vi "Main_DC.vi"() -> ()   [LabVIEW 2014]
uses:
  <vilib>/myRIO/Instrument Drivers/Utilities/Utilities.lvlib
  <vilib>/myRIO/Express VI/Onboard IO/Encoder/Encoder Express VI.xnode
  <vilib>/myRIO/Instrument Drivers/Onboard IO/Encoder/vis/Read.vi
  <vilib>/myRIO/Instrument Drivers/Onboard IO/Encoder/Encoder.lvlib
  <vilib>/myRIO/Common/Instrument Driver Framework/myRIO v1.0/Encoder/typedefs/Encoder Signal Mode.ctl
  <vilib>/myRIO/Common/Instrument Driver Framework/myRIO v1.0/Encoder/typedefs/Encoder Channels Enum.ctl
  <vilib>/myRIO/Common/Instrument Driver Framework/Utilities/typedefs/Generic FPGA Reference.ctl
  <vilib>/myRIO/Common/Instrument Driver Framework/Utilities/typedefs/myRIO v1.0 Reference.ctl
  <vilib>/myRIO/Common/Instrument Driver Framework/Utilities/typedefs/Hardware Version Enum.ctl
  <vilib>/myRIO/Common/Instrument Driver Framework/Utilities/typedefs/myRIO Generic Hardware Reference.ctl
  <vilib>/myRIO/Instrument Drivers/Onboard IO/Encoder/typedefs/Encoder Reference.ctl
  <vilib>/myRIO/Instrument Drivers/Onboard IO/Encoder/vis/myRIO Encoder Open.xnode
  <vilib>/myRIO/Common/Instrument Driver Framework/Utilities/vis/Is FPGA Ref Available.vi
  <vilib>/myRIO/Common/Instrument Driver Framework/myRIO v1.0/Encoder/vis/myRIO v1.1 Open Encoder.vi
  <vilib>/myRIO/Common/Instrument Driver Framework/myRIO v1.0/Encoder/vis/myRIO v1.0 Configure Encoder.vi
  <vilib>/myRIO/Common/Instrument Driver Framework/myRIO v1.0/Encoder/typedefs/Encoder Configuration v1.0.ctl
  <vilib>/userdefined/High Color/nirio_resource_hc.ctl
  <vilib>/myRIO/Common/Instrument Driver Framework/myRIO v1.0/Encoder/typedefs/Encoder Count Direction Enum.ctl
panel:
  in  "PWM freq [Hz]":dbl(slide)=10000.0 scale=5000.0..20000.0
  in  "PWM duty  [%]":dbl(slide) scale=-99.0..99.0
  in  "PWM duty  [%]":dbl(slide) scale=-99.0..99.0
  in  "PWM freq [Hz]":dbl(slide)=10000.0 scale=5000.0..20000.0
  in  "Reset Counter":bool
  out "Counter Direction":T1
  out "Counter Value":i32
  in  "[ESC]":bool
  # "DC Motor Testing"
  # "MOTOR 1"
  # "MOTOR 2"
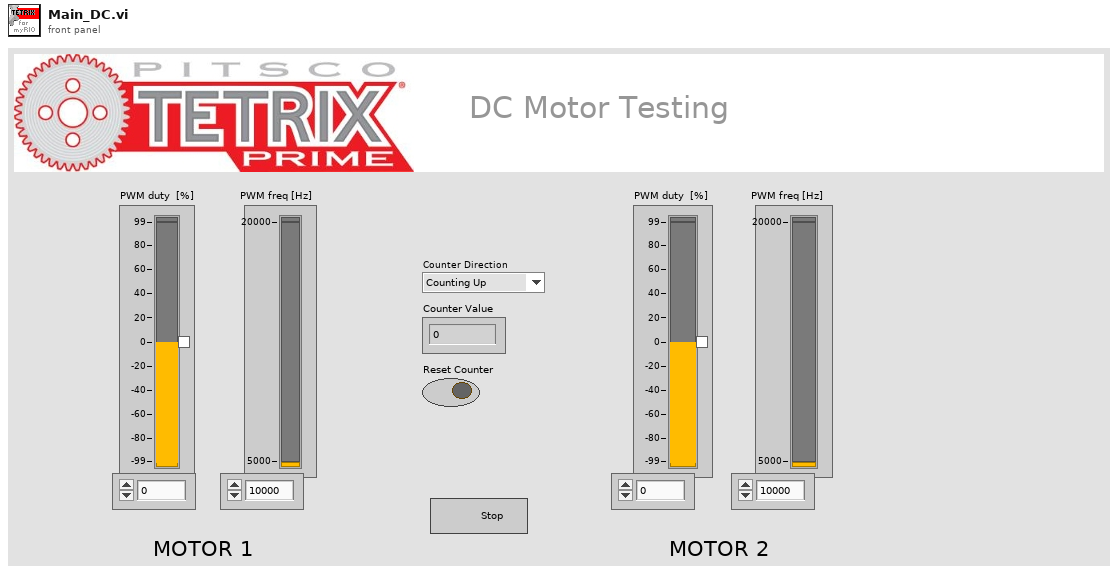
[diagram p1: front panel]
types:
  T1 = typedef "Encoder Count Direction Enum.ctl" = enum16{"Counting Up", "Counting Down"}
  T2 = typedef "Encoder.lvlib/Encoder Reference.ctl" = cluster{"myRIO Reference":T3, "Encoder Channels Enum":T7}
  T3 = typedef "myRIO Generic Hardware Reference.ctl" = cluster{"myRIO Model":T4, "myRIO Hardware Reference":T5}
  T4 = typedef "Hardware Version Enum.ctl" = enum16{"Unknown", "myRIO-1900", "myRIO-1950"}
  T5 = typedef "myRIO v1.0 Reference.ctl" = cluster{"Generic FPGA Reference":T6, "Allow multiple opens":bool}
  T6 = typedef "Generic FPGA Reference.ctl" = refnum<k20>
  T7 = typedef "Encoder Channels Enum.ctl" = enum16{"Not Connected", "C/ENC0", "C/ENC1", "A/ENC", "B/ENC"}
  T8 = typedef "Encoder Signal Mode.ctl" = enum16{"Quadrature phase signal", "Step and direction signal"}
  T9 = typedef "nirio_resource_hc.ctl" = tag
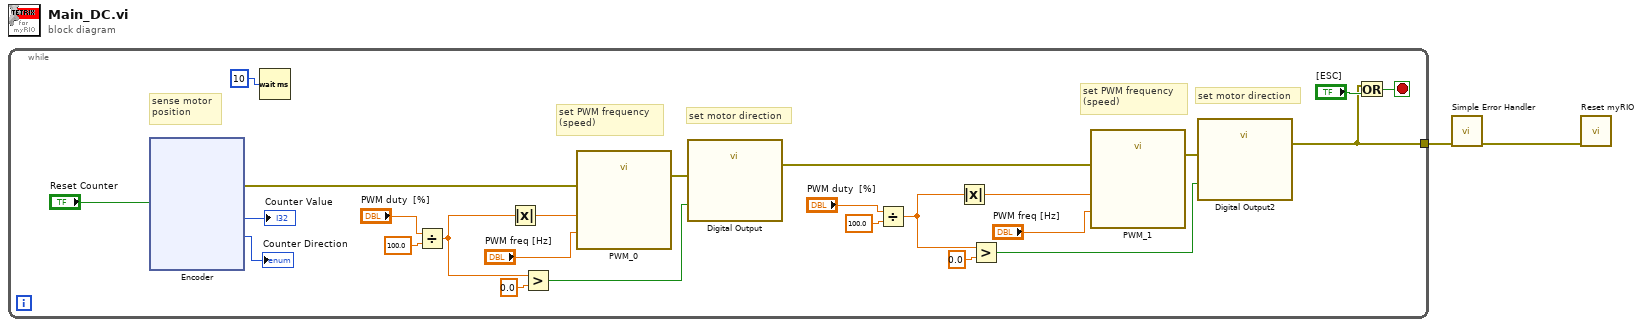
[diagram p0: block diagram]
diagram:
  n1 = while {
    tunnel: [w3] -> w1
    stop <- w27 stop-if-true
    # "set PWM frequency\n(speed)"
    # "set motor direction"
    # "sense motor \nposition"
    # "set PWM frequency\n(speed)"
    # "set motor direction"
    n2 = xnode "Encoder"("Reset Counter"="Reset Counter") -> ("Counter Value"=→"Counter Value":i32, "Counter Direction"=→"Counter Direction":enum16{"Counting Up", "Counting Down"}, "error out"=w24:errorcluster)  [unwired: 1 in, 1 out]
    n3 = Wait (ms)(milliseconds to wait=u32 10) -> ()  [unwired: 1 out]
    n4 = Divide(x="PWM duty  [%]", y=100.0) -> (x/y=w16:dbl)
    n5 = Absolute Value(x=w16) -> (abs(x)=w15:dbl)
    n6 = Greater?(x=w16, y=0.0) -> (0:w13:bool)
    n7 = call "PWM_0"("Duty Cycle (0-1)"=w15, "Frequency (Hz)"="PWM freq [Hz]", "error in (no error)"=w24) -> ("error out"=w23:errorcluster)  [unwired: 24 in]
    n8 = call "Digital Output"("A/DIO3 (Pin 17)"=w13, "error in (no error)"=w23) -> ("error out"=w5:errorcluster)  [unwired: 25 in]
    n9 = Divide(x="PWM duty  [%]", y=100.0) -> (x/y=w8:dbl)
    n10 = Absolute Value(x=w8) -> (abs(x)=w10:dbl)
    n11 = Greater?(x=w8, y=0.0) -> (0:w7:bool)
    n12 = call "PWM_1"("Duty Cycle (0-1)"=w10, "Frequency (Hz)"="PWM freq [Hz]", "error in (no error)"=w5) -> ("error out"=w4:errorcluster)  [unwired: 24 in]
    n13 = call "Digital Output2"("A/DIO2 (Pin 15)"=w7, "error in (no error)"=w4) -> ("error out"=w3:errorcluster)  [unwired: 25 in]
    n14 = Or(x=w3, y="[ESC]") -> (x .or. y?=w27:bool)
  }
  n15 = call <vilib>:"Simple Error Handler.vi"("error in (no error)"=w1) -> ("error out"=w2:errorcluster)  [unwired: 4 in, 4 out]
  n16 = call <vilib>:"Reset myRIO.vi"("error in (no error)"=w2) -> ()  [unwired: 10 in, 1 out]
